vi "Periodic Tasks.vi"(8 "error in":errorcluster) -> ()   [LabVIEW 2014]
doc: "This VI runs in parallel to other tasks. It can contain as many user-defined periodic loops as you need. These can carry out PID or other sorts of timed response."
uses:
  <vilib>/Rock Robotics/WPI/SafetyOutput/WPI_SafetyOutputConfigMenu.ctl
  <vilib>/Rock Robotics/WPI/Relay/WPI_RelayValue.ctl
  <vilib>/Rock Robotics/WPI/Joystick/WPI_JoystickGetSetRefNum.vi
  <vilib>/Rock Robotics/WPI/RobotDrive/WPI_RobotDriveGetSetRefNum.vi
  Global 2.vi
panel:
  out "Distance (Inches)":dbl
  out "Raw Voltage":dbl
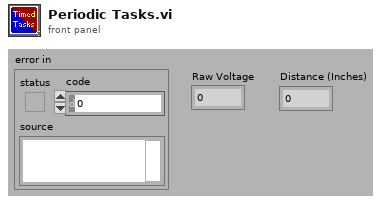
[diagram p1: front panel]
types:
  T1 = typedef "WPI_JoystickDevRef.ctl" = cluster{"Device":T2}
  T2 = typedef "WPI_JoystickDeviceEnum.ctl" = enum16{"USB 0", "USB 1", "USB 2", "USB 3", "USB 4", "USB 5"}
  T3 = typedef "WPI_RobotDriveDevRef.ctl" = cluster{"DevStatus":errorcluster, "Motors[]":T4[], "Square Inputs":bool, "Max Output":dbl}
  T4 = typedef "WPI_MotorControlDeviceRef.ctl" = cluster{"DeviceStatus":errorcluster, "Type":T5, "PWM":cluster{"Controller":T6, "PWM Channel":T7, "DeadBand":T8}, "CAN":cluster{"Device Number":u8, "Control Mode":T9, "Semaphore":T10, "Max Vout":dbl, "TalonSRX Control Mode":T11}, "Invert":bool, "TransformRef":T12, "InvTransformRef":T12}
  T5 = typedef "WPI_MotorControlType.ctl" = enum16{"PWM", "CAN", "CANTalonSRX"}
  T6 = typedef "FPGA_TypedefDigitalModule.ctl" = enum16{"Controller 1"}
  T7 = typedef "FPGA_DIOPWMChannel.ctl" = enum8{"PWM 0", "PWM 1", "PWM 2", "PWM 3", "PWM 4", "PWM 5", "PWM 6", "PWM 7", "PWM 8", "PWM 9", "PWM MXP 0", "PWM MXP 1", "PWM MXP 2", "PWM MXP 3", "PWM MXP 4", "PWM MXP 5", "PWM MXP 6", "PWM MXP 7", "PWM MXP 8", "PWM MXP 9", "Invalid"}
  T8 = typedef "WPI_PWMDeadband.ctl" = cluster{"Name":string, "maxPositivePwm":i32, "minPositivePwm":i32, "centerPwm":i32, "maxNegativePwm":i32, "minNegativePwm":i32, "angularRange":u16}
  T9 = typedef "WPI_CANJaguar_ControlMode.ctl" = enum8{"Percent VBus", "Current", "Speed", "Position", "Voltage"}
  T10 = typedef "Semaphore RefNum" = refnum<k1>
  T11 = typedef "WPI_CANTalonSRX_APIControlMode.ctl" = enum8{"Percent VBus", "Speed", "Position", "Slave", "Unchanged / Invalid"}
  T12 = typedef "WPI_PWMTransform_ConPane.ctl" = refnum<vi>
  T13 = cluster{"JoystickDevRef":T1, "RobotDriveDevRef":T3}
  T14 = typedef "WPI_RelayValue.ctl" = enum16{"Off", "On", "Forward", "Reverse"}
  T15 = typedef "WPI_RelayDevRef.ctl" = cluster{"DevStatus":errorcluster, "Relay Channel":T16, "Controller":T6, "Relay Direction":T17}
  T16 = typedef "FPGA_DIORelayChannel.ctl" = enum8{"Relay 0", "Relay 1", "Relay 2", "Relay 3", "Invalid"}
  T17 = typedef "WPI_RelayDirection.ctl" = enum16{"Both directions", "Forward only", "Reverse only"}
  T18 = typedef "WPI_SafetyOutputConfigMenu.ctl" = enum16{"Enable", "Disable"}
  T19 = typedef "WPI_AnalogChannelDevRef.ctl" = cluster{"DevStatus":errorcluster, "Controller":T20, "Analog Channel":T21}
  T20 = typedef "FPGA_TypedefAnalogModule.ctl" = enum16{"Controller 1"}
  T21 = typedef "FPGA_AIChannel.ctl" = enum8{"AI 0", "AI 1", "AI 2", "AI 3", "AI MXP 0", "AI MXP 1", "AI MXP 2", "AI MXP 3", "Invalid"}
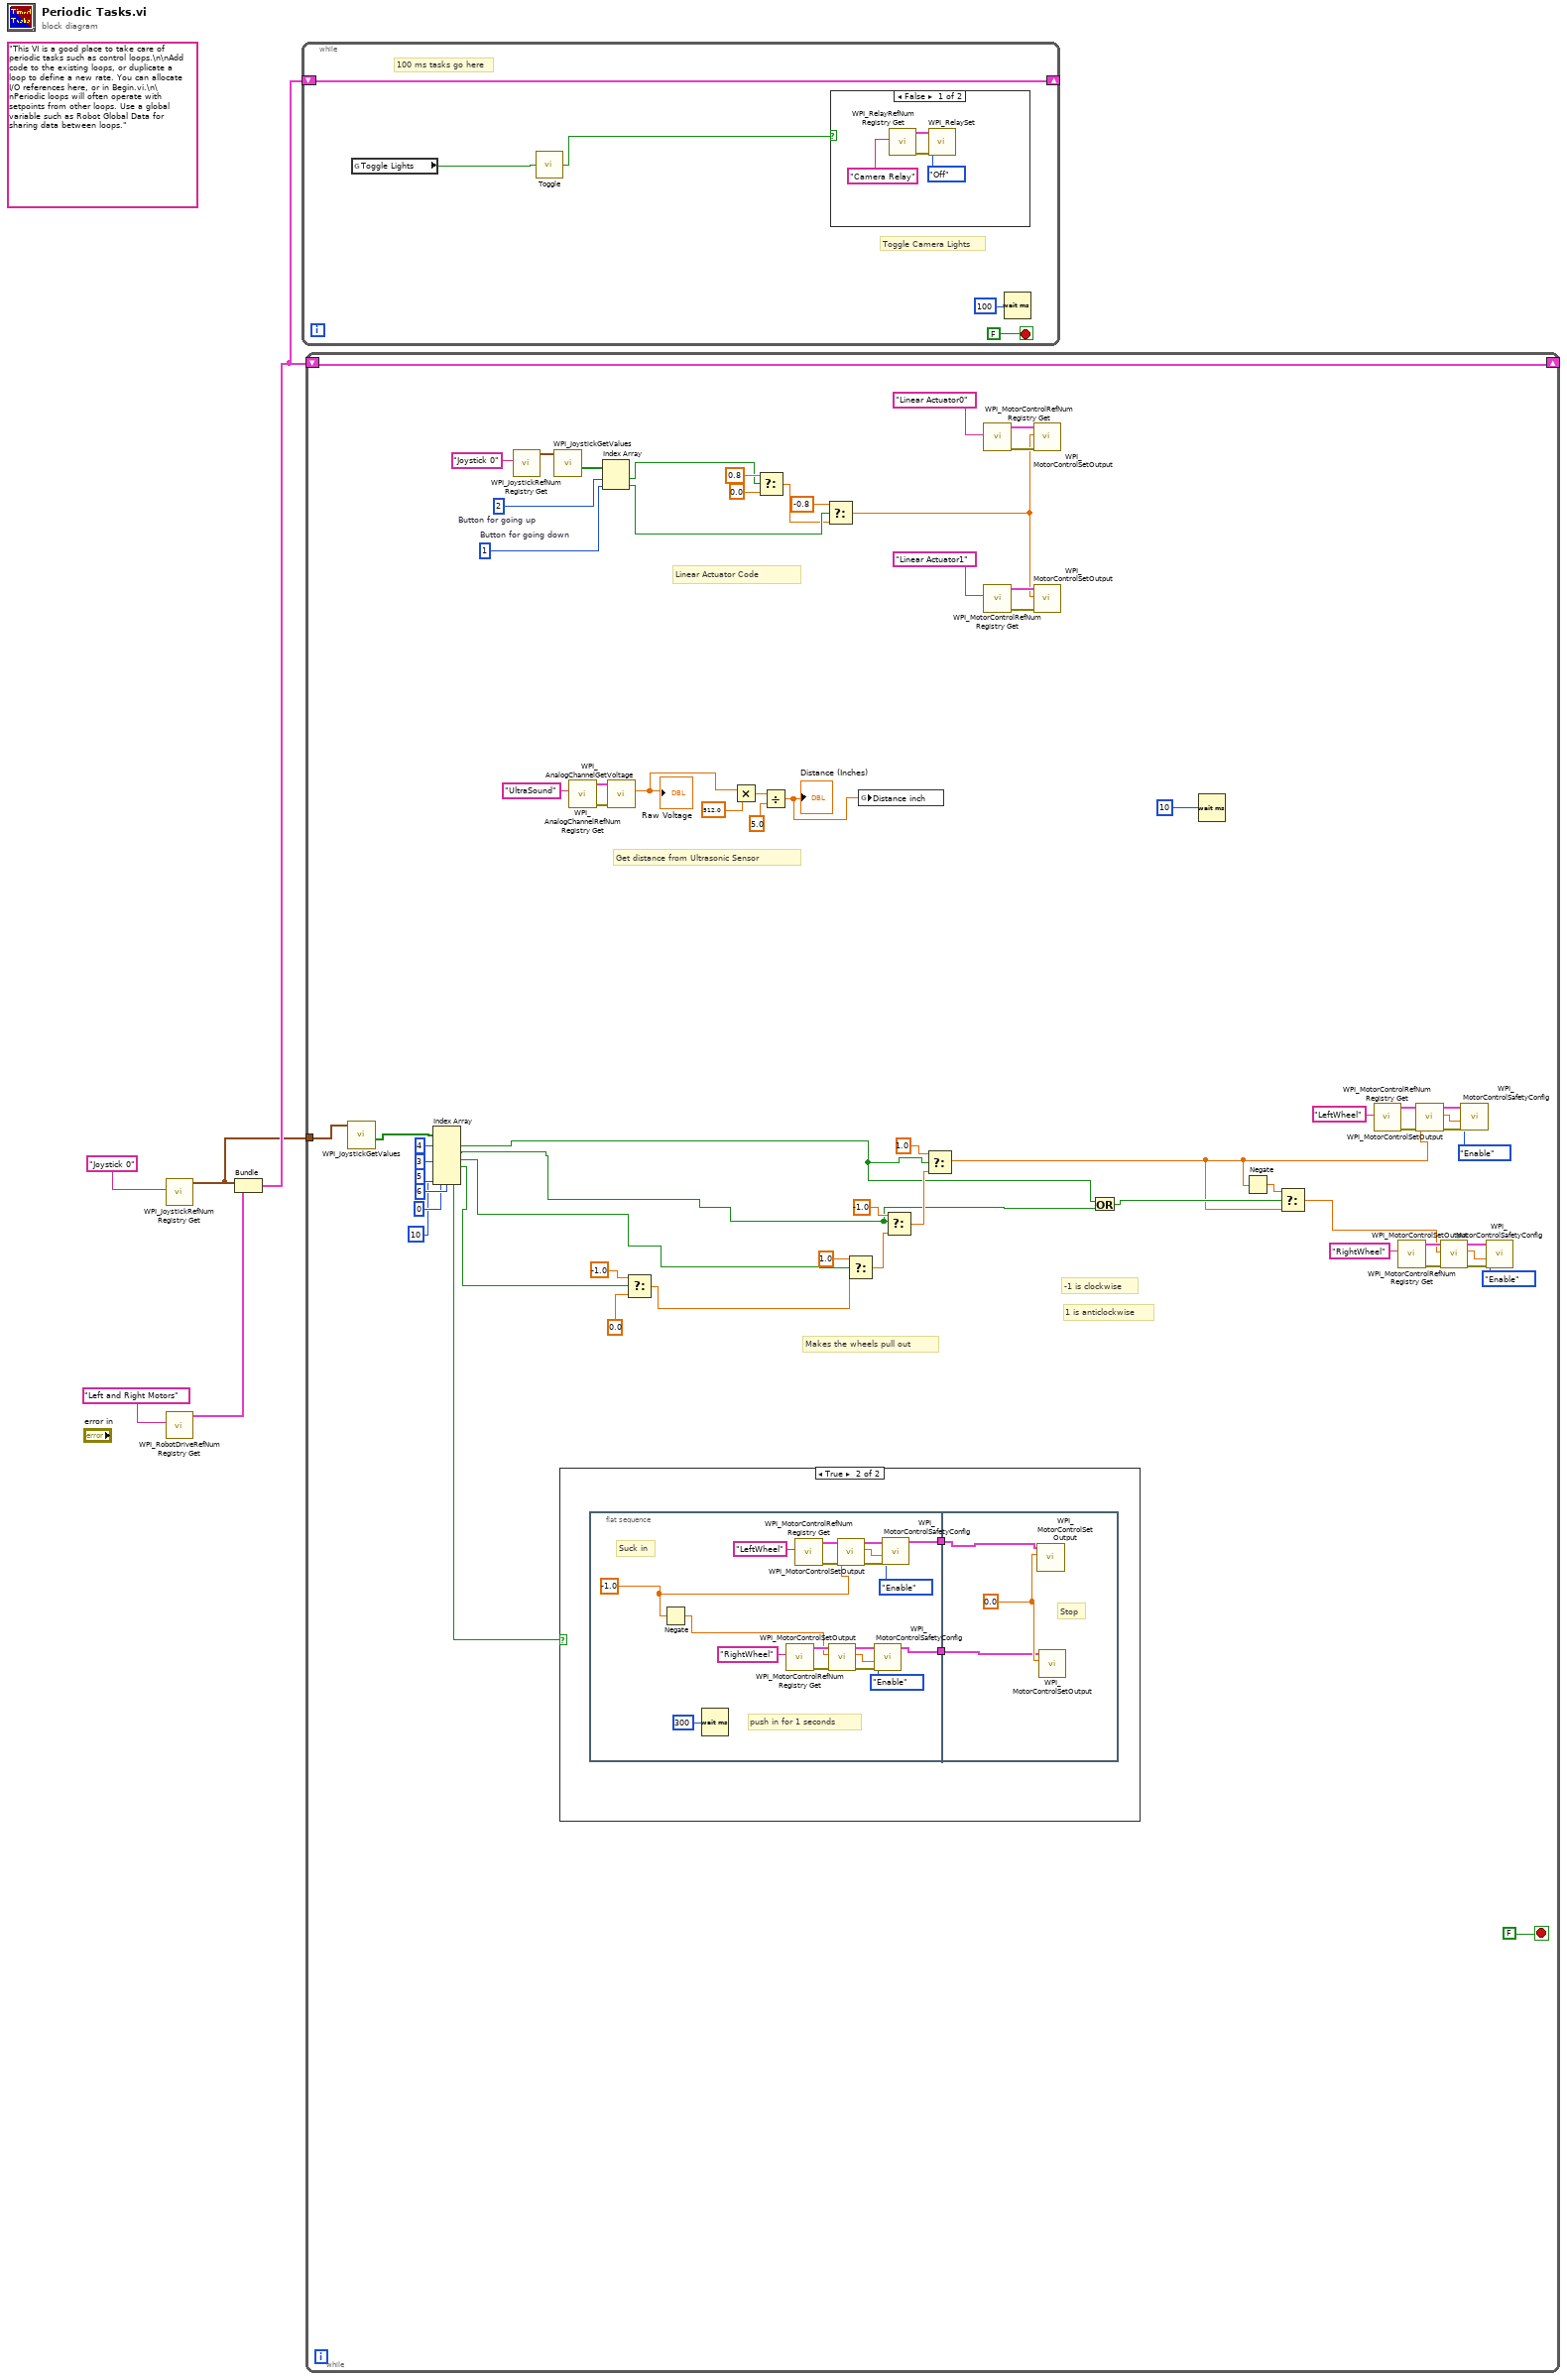
[diagram p0: block diagram]
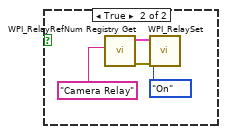
[diagram p3: hidden frame]
diagram:
  (unwired) "This VI is a good place to take care of periodic tasks such as control loops.\n\nAdd code to the existing loops, or duplicate a loop to define a new rate. You can allocate I/O references here, or in Begin.vi.\n\nPeriodic loops will often operate with setpoints from other loops. Use a global variable such as Robot Global Data for sharing data between loops."
  n1 = call <vilib>:"WPI_JoystickRefNum Registry Get.vi"("refnum name"="Joystick 0") -> ("JoystickDevRef"=w1:T1)  [unwired: 1 in, 9 out]
  n2 = call <vilib>:"WPI_RobotDriveRefNum Registry Get.vi"("refnum name"="Left and Right Motors") -> ("RobotDriveDevRef"=w3:T3)  [unwired: 1 in, 9 out]
  n3 = Bundle("JoystickDevRef"=w1, "RobotDriveDevRef"=w3) -> (w2:T13)  [unwired: 1 out]
  n4 = while {
    shift-right: [w8] -> _
    shift-left: w2 -> [w8]
    stop <- FALSE stop-if-true
    # "Toggle Camera Lights"
    # "100 ms tasks go here"
    n5 = global read "Global 2.vi" "Toggle Lights"() -> (w7:bool)
    n6 = call "Toggle.vi"("Input"=w7) -> ("Output"=w6:bool)
    n7 = case shown="False" w6 {
      frame False {
        n8 = call <vilib>:"WPI_RelayRefNum Registry Get.vi"("refnum name"="Camera Relay") -> ("error out"=w13:errorcluster, "RelayDevRef"=w12:T15)  [unwired: 9 in]
        n9 = call <vilib>:"WPI_RelaySet.vi"("error in (no error)"=w13, "RelayValue"=WPI_RelayValue."Off", "RelayDevRef"=w12) -> ()  [unwired: 7 in, 2 out]
      }
      frame True {
        n10 = call <vilib>:"WPI_RelayRefNum Registry Get.vi"("refnum name"="Camera Relay") -> ("error out"=w17:errorcluster, "RelayDevRef"=w16:T15)  [unwired: 9 in]
        n11 = call <vilib>:"WPI_RelaySet.vi"("error in (no error)"=w17, "RelayValue"=WPI_RelayValue."On", "RelayDevRef"=w16) -> ()  [unwired: 7 in, 2 out]
      }
    }
    n12 = Wait (ms)(milliseconds to wait=u32 100) -> ()  [unwired: 1 out]
  }
  n13 = while {
    shift-right: [w84] -> _
    shift-left: w2 -> [w84]
    tunnel: w1 -> [w23]
    stop <- FALSE stop-if-true
    w79 = 1  # Button for going down
    w80 = 2  # Button for going up
    # "1 is anticlockwise"
    # "-1 is clockwise"
    # "Makes the wheels pull out"
    # "Get distance from Ultrasonic Sensor"
    # "Linear Actuator Code"
    n14 = call <vilib>:"WPI_JoystickGetValues.vi"("JoystickDevRef"=w23) -> ("Buttons"=w22:bool[])  [unwired: 6 in, 4 out]
    n15 = Index Array(array=w22, index #1=4 ("index"), index #2=3 ("index"), index #3=5 ("index"), index #4=6 ("index"), index #5=0 ("index"), index #6=10 ("index")) -> (element #1=w24:bool, element #2=w25:bool, element #3=w26:bool, element #4=w30:bool, element #5=w20:bool)  [unwired: 1 out]
    n16 = call <vilib>:"WPI_JoystickRefNum Registry Get.vi"("refnum name"="Joystick 0") -> ("JoystickDevRef"=w82:T1)  [unwired: 9 in, 1 out]
    n17 = call <vilib>:"WPI_JoystickGetValues.vi"("JoystickDevRef"=w82) -> ("Buttons"=w81:bool[])  [unwired: 6 in, 4 out]
    n18 = case shown="True" w20 {
      frame False {
      }
      frame True {
        n19 = flat-sequence {
          tunnel: [w90] -> w88
          tunnel: [w89] -> w87
          tunnel: w88 -> [w108]
          tunnel: w87 -> [w109]
          frame #0 {
            w92 = -1.0
            # "Suck in"
            # "push in for 1 seconds"
            n20 = Negate(x=w92) -> (-x=w93:dbl)
            n21 = Wait (ms)(milliseconds to wait=u32 300) -> ()  [unwired: 1 out]
            n22 = call <vilib>:"WPI_MotorControlRefNum Registry Get.vi"("refnum name"="RightWheel") -> ("error out"=w105:errorcluster, "MotorControlDevRef"=w104:T4)  [unwired: 9 in]
            n23 = call <vilib>:"WPI_MotorControlRefNum Registry Get.vi"("refnum name"="LeftWheel") -> ("error out"=w107:errorcluster, "MotorControlDevRef"=w106:T4)  [unwired: 9 in]
            n24 = call <vilib>:"WPI_MotorControlSetOutput.vi"("error in (no error)"=w105, "Output"=w93, "MotorControlDevRef"=w104) -> ("error out"=w98:errorcluster, "Motor Output"=w97:dbl, "MotorControlDevRef"=w96:T4)  [unwired: 6 in]
            n25 = call <vilib>:"WPI_MotorControlSetOutput.vi"("error in (no error)"=w107, "Output"=w92, "MotorControlDevRef"=w106) -> ("error out"=w101:errorcluster, "Motor Output"=w100:dbl, "MotorControlDevRef"=w99:T4)  [unwired: 6 in]
            n26 = call <vilib>:"WPI_MotorControlSafetyConfig.vi"("error in (no error)"=w98, "timeout (s)"=w97, "mode"=WPI_SafetyOutputConfigMenu."Enable", "MotorControlDevRef"=w96) -> ("MotorControlDevRef"=w90:T4)  [unwired: 6 in, 1 out]
            n27 = call <vilib>:"WPI_MotorControlSafetyConfig.vi"("error in (no error)"=w101, "timeout (s)"=w100, "mode"=WPI_SafetyOutputConfigMenu."Enable", "MotorControlDevRef"=w99) -> ("MotorControlDevRef"=w89:T4)  [unwired: 6 in, 1 out]
          }
          frame #1 {
            w110 = 0.0
            # "Stop"
            n28 = call <vilib>:"WPI_MotorControlSetOutput.vi"("Output"=w110, "MotorControlDevRef"=w109) -> ()  [unwired: 7 in, 3 out]
            n29 = call <vilib>:"WPI_MotorControlSetOutput.vi"("Output"=w110, "MotorControlDevRef"=w108) -> ()  [unwired: 7 in, 3 out]
          }
        }
      }
    }
    n30 = call <vilib>:"WPI_AnalogChannelRefNum Registry Get.vi"("refnum name"="UltraSound") -> ("error out"=w64:errorcluster, "AIDeviceRef"=w63:T19)  [unwired: 9 in]
    n31 = Index Array(array=w81, index #1=w80, index #2=w79) -> (element #1=w71:bool, element #2=w72:bool)
    n32 = call <vilib>:"WPI_AnalogChannelGetVoltage.vi"("error in (no error)"=w64, "AIDeviceRef"=w63) -> ("Voltage"=w62:dbl)  [unwired: 7 in, 2 out]
    "Raw Voltage" <- w62
    n33 = Select(t=-1.0, s=w30, f=0.0) -> (s? t:f=w27:dbl)
    n34 = Multiply(x=w62, y=512.0) -> (x*y=w60:dbl)
    n35 = Select(t=0.8, s=w71, f=0.0) -> (s? t:f=w70:dbl)
    n36 = Divide(x=w60, y=5.0) -> (x/y=w58:dbl)
    "Distance (Inches)" <- w58
    n37 = Select(t=-0.8, s=w72, f=w70) -> (s? t:f=w66:dbl)
    n38 = Select(t=1.0, s=w26, f=w27) -> (s? t:f=w40:dbl)
    n39 = global write "Global 2.vi" "Distance inch"(w58) -> ()
    n40 = Select(t=-1.0, s=w25, f=w40) -> (s? t:f=w41:dbl)
    n41 = Select(t=1.0, s=w24, f=w41) -> (s? t:f=w35:dbl)
    n42 = call <vilib>:"WPI_MotorControlRefNum Registry Get.vi"("refnum name"="Linear Actuator0") -> ("error out"=w78:errorcluster, "MotorControlDevRef"=w77:T4)  [unwired: 9 in]
    n43 = call <vilib>:"WPI_MotorControlRefNum Registry Get.vi"("refnum name"="Linear Actuator1") -> ("error out"=w69:errorcluster, "MotorControlDevRef"=w68:T4)  [unwired: 9 in]
    n44 = call <vilib>:"WPI_MotorControlSetOutput.vi"("error in (no error)"=w78, "Output"=w66, "MotorControlDevRef"=w77) -> ()  [unwired: 6 in, 3 out]
    n45 = call <vilib>:"WPI_MotorControlSetOutput.vi"("error in (no error)"=w69, "Output"=w66, "MotorControlDevRef"=w68) -> ()  [unwired: 6 in, 3 out]
    n46 = Or(x=w24, y=w25) -> (x .or. y?=w37:bool)
    n47 = Wait (ms)(milliseconds to wait=u32 10) -> ()  [unwired: 1 out]
    n48 = Negate(x=w35) -> (-x=w36:dbl)
    n49 = Select(t=w36, s=w37, f=w35) -> (s? t:f=w38:dbl)
    n50 = call <vilib>:"WPI_MotorControlRefNum Registry Get.vi"("refnum name"="LeftWheel") -> ("error out"=w56:errorcluster, "MotorControlDevRef"=w55:T4)  [unwired: 9 in]
    n51 = call <vilib>:"WPI_MotorControlRefNum Registry Get.vi"("refnum name"="RightWheel") -> ("error out"=w54:errorcluster, "MotorControlDevRef"=w53:T4)  [unwired: 9 in]
    n52 = call <vilib>:"WPI_MotorControlSetOutput.vi"("error in (no error)"=w56, "Output"=w35, "MotorControlDevRef"=w55) -> ("error out"=w50:errorcluster, "Motor Output"=w49:dbl, "MotorControlDevRef"=w48:T4)  [unwired: 6 in]
    n53 = call <vilib>:"WPI_MotorControlSetOutput.vi"("error in (no error)"=w54, "Output"=w38, "MotorControlDevRef"=w53) -> ("error out"=w47:errorcluster, "Motor Output"=w46:dbl, "MotorControlDevRef"=w45:T4)  [unwired: 6 in]
    n54 = call <vilib>:"WPI_MotorControlSafetyConfig.vi"("error in (no error)"=w50, "timeout (s)"=w49, "mode"=WPI_SafetyOutputConfigMenu."Enable", "MotorControlDevRef"=w48) -> ()  [unwired: 6 in, 2 out]
    n55 = call <vilib>:"WPI_MotorControlSafetyConfig.vi"("error in (no error)"=w47, "timeout (s)"=w46, "mode"=WPI_SafetyOutputConfigMenu."Enable", "MotorControlDevRef"=w45) -> ()  [unwired: 6 in, 2 out]
  }
